vi "WinCI Rename.vi"(8 "error in (no error)":errorcluster, 9 "new filename":path, 10 "current filename":path, 11 "source control reference in":T1) -> (0 "error out":errorcluster, 2 "status message":string, 3 "source control reference out":T1)   [LabVIEW 2020, in "NI_SCC_WinCI.lvlib"]
uses:
  <vilib>/SourceControl/Providers/WinCI/NI_SCC_WinCI.lvlib
  <vilib>/SourceControl/sccapi/SCCAPI Refnum.ctl
  <vilib>/SourceControl/support/SCCSup Message Strings GLBL.vi
  <vilib>/SourceControl/sccapi/NI_SCC.lvlib
panel:
  out "result":i32
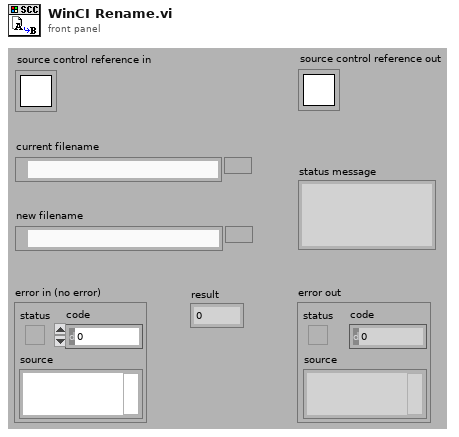
[diagram p1: front panel]
types:
  T1 = typedef "NI_SCC.lvlib/SCCAPI Refnum.ctl" = refnum<k1>
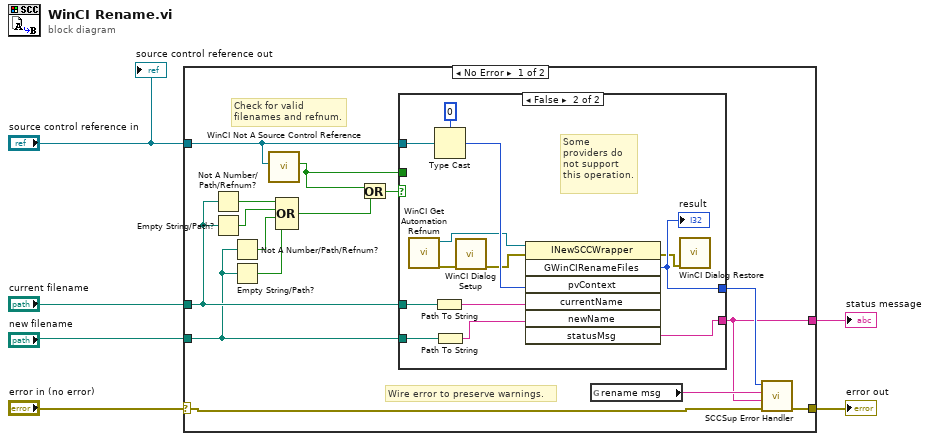
[diagram p0: block diagram]
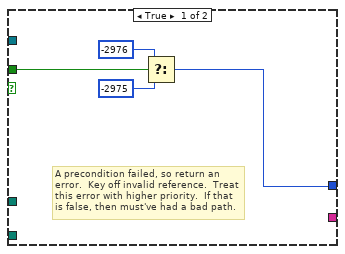
[diagram p2: hidden frame]
diagram:
  n1 = case shown="No Error" "error in (no error)" {
    selector: "error in (no error)" -> [w17 w39]
    tunnel: [w21 w39] -> w5
    tunnel: "source control reference in" -> [w8 _]
    tunnel: [w18 _] -> w3
    tunnel: "current filename" -> [w13 _]
    tunnel: "new filename" -> [w11 _]
    frame No Error {
      # "Check for valid filenames and refnum."
      # "Wire error to preserve warnings."
      n2 = Not A Number/Path/Refnum?(number/path/refnum=w13) -> (NaN/Path/Refnum?=w14:bool)
      n3 = Empty String/Path?(string/path=w13) -> (empty?=w15:bool)
      n4 = Not A Number/Path/Refnum?(number/path/refnum=w11) -> (NaN/Path/Refnum?=w10:bool)
      n5 = Empty String/Path?(string/path=w11) -> (empty?=w9:bool)
      n6 = call <vilib>:"WinCI Not A Source Control Reference.vi"("source control reference in"=w8) -> ("not a source control reference?"=w7:bool)  [unwired: 1 in, 9 out]
      n7 = Compound Arithmetic op=OR(w14, w15, w10, w9) -> (w16:bool)
      n8 = Or(x=w7, y=w16) -> (x .or. y?=w12:bool)
      n9 = case shown="False" w12 {
        tunnel: w8 -> [_ w38]
        tunnel: [_ w33] -> w18
        tunnel: w13 -> [_ w36]
        tunnel: w11 -> [_ w35]
        tunnel: [w22 w34] -> w20
        tunnel: w7 -> [w23 _]
        frame True {
          # "A precondition failed, so return an error.  Key off invalid reference.  Treat this error with higher priority.  If that is false, then must've had a bad path."
          n10 = Select(t=-2976 ("result"), s=w23, f=-2975 ("result")) -> (s? t:f=w22:i32)
        }
        frame False {
          # "Some providers do not support this operation."
          n11 = call <vilib>:"WinCI Get Automation Refnum.vi"() -> ("error out"=w28:errorcluster, "automation refnum"=w29:refnum<k7>)  [unwired: 10 out]
          n12 = Path To String(path=w36) -> (string=w31:string)
          n13 = Type Cast(type=u32 0, x=w38) -> (*(type *) &x=w30:u32)
          n14 = Path To String(path=w35) -> (string=w32:string)
          n15 = call <vilib>:"WinCI Dialog Setup.vi"("error in"=w28) -> ("error out"=w27:errorcluster)  [unwired: 10 out]
          n16 = invoke class="INewSCCWrapper" method="GWinCIRenameFiles"(reference=w29, error in=w27, "pvContext"=w30, "currentName"=w31, "newName"=w32) -> (error out=w26:errorcluster, "GWinCIRenameFiles"=w34:i32, "statusMsg"=w33:string)  [unwired: 2 in, 4 out]
          "result" <- w34
          n17 = call <vilib>:"WinCI Dialog Restore.vi"("error in"=w26) -> ()  [unwired: 11 out]
        }
      }
      n18 = global read "SCCSup Message Strings GLBL.vi" "rename msg"() -> (w19:string)
      n19 = call <vilib>:"SCCSup Error Handler.vi"("error in (no error)"=w17, "additional message"=w18, "operation message"=w19, "scc error code"=w20) -> ("error out"=w21:errorcluster)  [unwired: 7 out]
    }
    frame Error {
    }
  }
  "error out" <- w5
  "status message" <- w3
  "source control reference out" <- "source control reference in"
